vi "calibrateEvent.vi"(8 "error in (no error)":errorcluster, 11 "rf in":refnum<class "rf.lvclass">) -> (0 "error out":errorcluster, 3 "rf out":refnum<class "rf.lvclass">)   [LabVIEW 2009, in "Tools.lvlib" / "Scripting.lvlib" / "rf.lvclass"]
uses:
  rf.lvclass
  rf.lvclass/rf.ctl
  ScriptEvent.lvclass
  DatabaseHelpers/Database Objects/Channel/RfOutputChannel/RfOutputChannel.lvclass
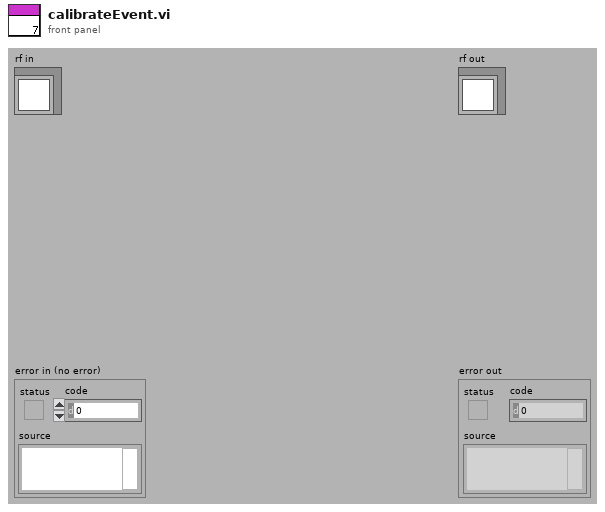
[diagram p1: front panel]
types:
  T1 = cluster{"frequency":cluster{"gradient":dbl, "offset":dbl}, "amplitude":cluster{"gradient":dbl, "offset":dbl}, "phase":cluster{"gradient":dbl, "offset":dbl}}
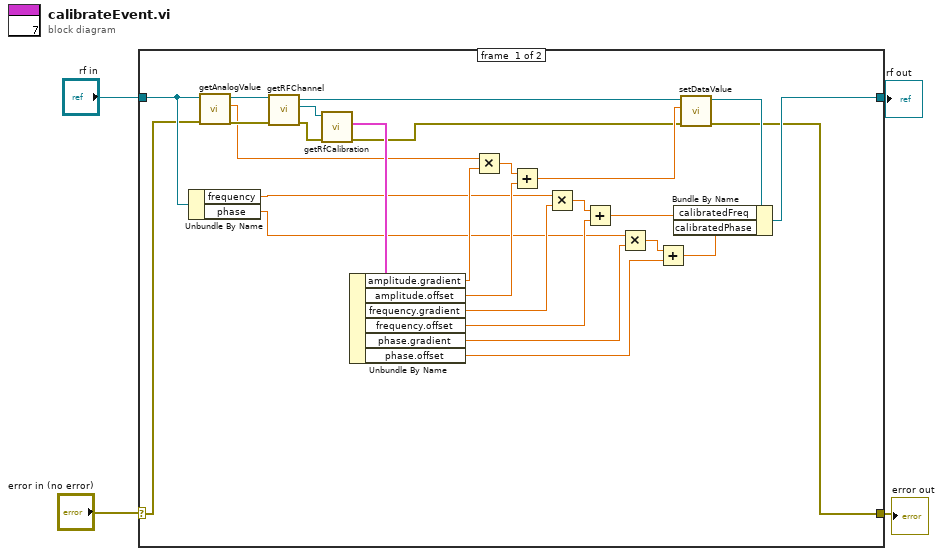
[diagram p0: block diagram]
diagram:
  n1 = case shown="No Error" "error in (no error)" {
    selector: "error in (no error)" -> [w30 w33]
    tunnel: "rf in" -> [w31 w32]
    tunnel: [w5 w33] -> w2
    tunnel: [w10 w32] -> w1
    frame #0 {
      n2 = Unbundle By Name(w31) -> ("frequency"=w19:dbl, "phase"=w15:dbl)
      n3 = call "getAnalogValue.vi"("error in (no error)"=w30, "ScriptEvent in"=w31) -> ("error out"=w28:errorcluster, "analogValue"=w24:dbl, "ScriptEvent out"=w29:refnum<class "rf.lvclass">)  [unwired: 7 in]
      n4 = call "getRFChannel.vi"("error in (no error)"=w28, "rf.lvclass in"=w29) -> ("error out"=w26:errorcluster, "RfOutputChannel.lvclass"=w27:refnum<class "RfOutputChannel.lvclass">, "rf.lvclass out"=w8:refnum<class "rf.lvclass">)  [unwired: 7 in]
      n5 = call "getRfCalibration.vi"("error in (no error)"=w26, "RfOutputChannel in"=w27) -> ("error out"=w6:errorcluster, "calibration"=w25:T1)  [unwired: 7 in, 1 out]
      n6 = Unbundle By Name(w25) -> ("amplitude.gradient"=w23:dbl, "amplitude.offset"=w21:dbl, "frequency.gradient"=w18:dbl, "frequency.offset"=w17:dbl, "phase.gradient"=w14:dbl, "phase.offset"=w13:dbl)
      n7 = Multiply(x=w24, y=w23) -> (x*y=w22:dbl)
      n8 = Add(x=w22, y=w21) -> (x+y=w7:dbl)
      n9 = Multiply(x=w19, y=w18) -> (x*y=w20:dbl)
      n10 = Add(x=w20, y=w17) -> (x+y=w12:dbl)
      n11 = Multiply(x=w15, y=w14) -> (x*y=w16:dbl)
      n12 = Add(x=w16, y=w13) -> (x+y=w11:dbl)
      n13 = call "setDataValue.vi"("error in (no error)"=w6, "dataValue"=w7, "ScriptEvent.lvclass in"=w8) -> ("error out"=w5:errorcluster, "ScriptEvent.lvclass out"=w9:refnum<class "rf.lvclass">)  [unwired: 7 in]
      n14 = Bundle By Name(cluster=w9, "calibratedFreq"=w12, "calibratedPhase"=w11) -> (w10:refnum<class "rf.lvclass">)
    }
    frame #1 {
    }
  }
  "error out" <- w2
  "rf out" <- w1
